vi "FPGAController_v5.1.vi"() -> ()   [LabVIEW 2015]
uses:
  Detector_Cluster.ctl
  <vilib>/Utility/miscctls.llb/LVPointTypeDef.ctl
  <vilib>/FPGAPlugInAG/PXIe-7971R/niLvFpga_Open_PXIe-7971R.vi
  <userlib>/_OpenG.lib/comparison/comparison.llb/Variant Changed__ogtk.vi
  <vilib>/Utility/error.llb/Error Cluster From Error Code.vi
  <vilib>/rvi/errors/niLvFpgaAdjustHostInterfaceError.vi
  <vilib>/FPGAPlugInAG/PXIe-7971R/niLvFpga_Close_PXIe-7971R.vi
  <vilib>/rvi/interface/nirviOpenFPGA/nirviOpenFPGA.xnode
  FPGA Bitfiles/FPGA2_FPGATarget_FPGAcode2.1_u+OfLr1fgUM.lvbitx
  <vilib>/rvi/interface/nirviReadWriteControl/nirviReadWriteControl.xnode
  Limits_In.ctl
  <vilib>/rvi/interface/nirviCloseFPGA/nirviCloseFPGA.xnode
  NiFpgaLv.dll
panel:
  in  "Trigger String 2":string="Disarm Trigger"
  in  "Trigger String 1":string="Rearm Trigger"
  in  "Tab Control":enum32{"IO/Control", "Error Management"}(tab)
  out "Trigger Armed":bool
  in  "Arm Trigger":bool
  in  "One Shot Mode":bool
  in  "Auto Threshold":bool
  in  "Sensitivity":dbl=1.2 step=0.2 format="%_3g"
  in  "Filter Thresholds":T1={"1"=887988, "2"=361992, "3"=138762, "4"=54306, "5"=41730, "6"=29358, "7"=21165}
  in  "error in (no error)":errorcluster
  out "error out":errorcluster
  out "Runtime Error":errorcluster
  out "Updating PSU":bool
  in  "stop":bool
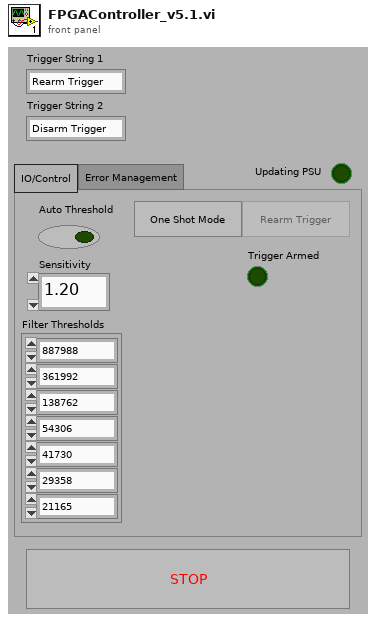
[diagram p1: front panel]
types:
  T1 = typedef "Detector_Cluster.ctl" = cluster{"1":i32, "2":i32, "3":i32, "4":i32, "5":i32, "6":i32, "7":i32}
  T2 = enum8{"Enabled", "Disabled", "Disabled and Grayed Out"}
  T3 = typedef "LVPointTypeDef.ctl" = cluster{"Horizontal":i16, "Vertical":i16}
  T4 = typedef "Limits_In.ctl" = cluster{"High Charge Limit":i16, "Low Charge Limit":i16, "High Velocity Count":i32, "Low Velocity Count":i32, "High Mass Limit":i64, "Low Mass Limit":i64}
  T5 = cluster{"1":dbl, "2":dbl, "3":dbl, "4":dbl, "5":dbl, "6":dbl, "7":dbl}
  T6 = cluster{"1":i16, "2":i16, "3":i16, "4":i16, "5":i16, "6":i16, "7":i16}
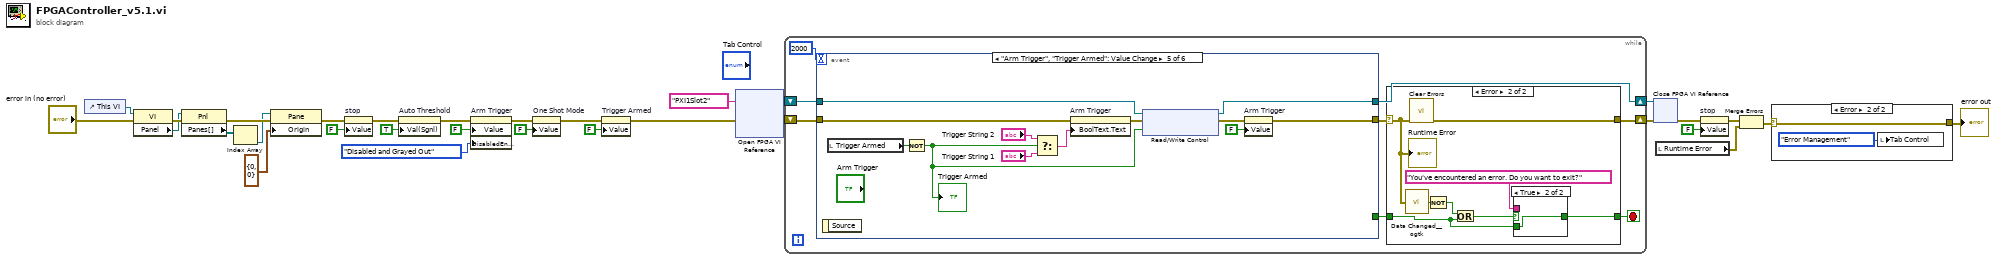
[diagram p0: block diagram]
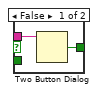
[diagram p4: hidden frame]
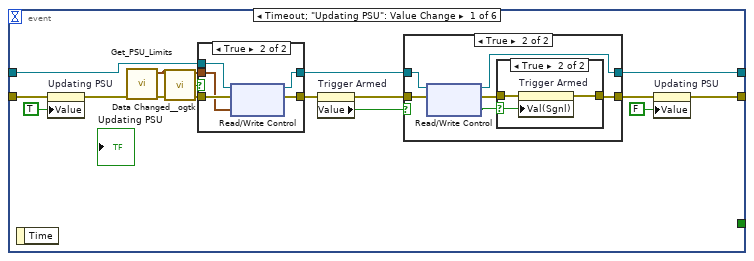
[diagram p5: hidden frame]
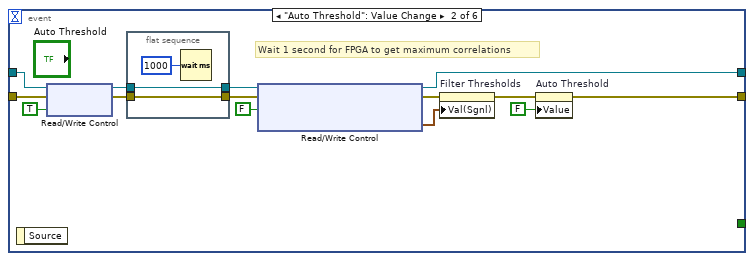
[diagram p9: hidden frame]
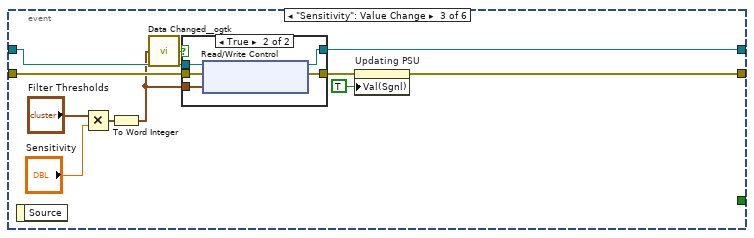
[diagram p10: hidden frame]
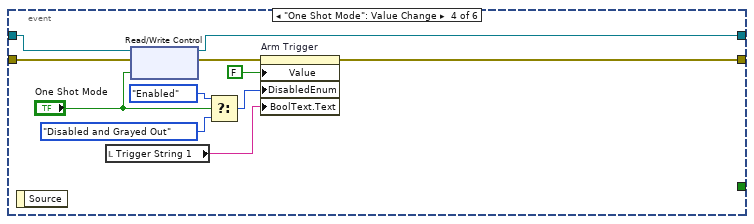
[diagram p12: hidden frame]
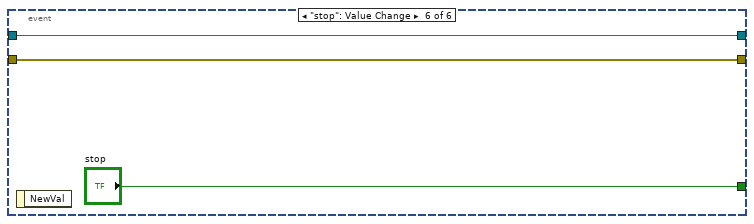
[diagram p13: hidden frame]
diagram:
  n1 = control-ref of="This VI"() -> (w31:refnum<vi>)
  n2 = property class="VI"(reference=w31, error in="error in (no error)") -> (error out=w30:errorcluster, "Panel"=w29:refnum<vi>)  [unwired: 1 out]
  n3 = property class="Pnl"(reference=w29, error in=w30) -> (error out=w28:errorcluster, "Panes[]"=w27:refnum<vi>[])  [unwired: 1 out]
  n4 = Index Array(array=w27) -> (element=w26:refnum<vi>)  [unwired: 1 in]
  n5 = property class="Pane"(reference=w26, error in=w28, "Origin"=T3 {"Horizontal"=0, "Vertical"=0}) -> (error out=w19:errorcluster)  [unwired: 1 out]
  n6 = property on="stop" class="Bool (strict)"(error in=w19, "Value"=FALSE ("stop")) -> (error out=w15:errorcluster)  [unwired: 1 in, 1 out]
  n7 = property on="Auto Threshold" class="Bool (strict)"(error in=w15, "Val(Sgnl)"=TRUE ("Value (Signaling)")) -> (error out=w7:errorcluster)  [unwired: 1 in, 1 out]
  n8 = property on="Arm Trigger" class="Bool (strict)"(error in=w7, "Value"=FALSE ("Arm Trigger"), "DisabledEnum"=T2."Disabled and Grayed Out" ("Disabled")) -> (error out=w5:errorcluster)  [unwired: 1 in, 1 out]
  n9 = property on="One Shot Mode" class="Bool (strict)"(error in=w5, "Value"=FALSE ("One Shot Mode")) -> (error out=w3:errorcluster)  [unwired: 1 in, 1 out]
  n10 = property on="Trigger Armed" class="Bool (strict)"(error in=w3, "Value"=FALSE ("Armed")) -> (error out=w1:errorcluster)  [unwired: 1 in, 1 out]
  n11 = xnode "Open FPGA VI Reference"("error in"=w1, "resource name"=tag "PXI1Slot2") -> ("FPGA VI Reference Out"=w23:refnum<k20>, "error out"=w21:errorcluster)
  n12 = while {
    shift-right: [w32] -> w20
    shift-left: w21 -> [w38]
    shift-right: [w36] -> w22
    shift-left: w23 -> [w37]
    stop <- w34 stop-if-true
    n13 = event shown="[4] \"Arm Trigger\", \"Trigger Armed\": Value Change" {
      selector: _ -> [_ _ _ _ _ _]
      dyn-events: _ -> [_ _ _ _ _ _]
      timeout: 2000 -> [_ _ _ _ _ _]
      tunnel: [_ _ _ _ _ "stop"] -> w33
      tunnel: w38 -> [w65 w98 w113 w132 w144 w146]
      tunnel: [w59 w100 w107 w124 w134 w146] -> w35
      tunnel: w37 -> [w67 w97 w114 w131 w139 w145]
      tunnel: [w54 w92 w110 w123 w138 w145] -> w36
      event Timeout; "Updating PSU": Value Change {
        n14 = event-data() -> ()  [unwired: 1 in, 1 out]
        n15 = property on="Updating PSU" class="Bool (strict)"(error in=w65, "Value"=TRUE ("Updating PSU")) -> (error out=w62:errorcluster)  [unwired: 1 in, 1 out]
        n16 = call "Get_PSU_Limits.vi"("error in (no error)"=w62) -> ("error out"=w66:errorcluster, "Limits"=w61:T4)  [unwired: 9 in]
        n17 = call-poly <userlib>:"Data Changed__ogtk.vi"("Variant"=w61) -> ("Changed"=w60:bool)
        n18 = case shown="True" w60 {
          tunnel: w67 -> [w81 w86]
          tunnel: w66 -> [w80 w85]
          tunnel: [w81 w84] -> w55
          tunnel: [w80 w83] -> w58
          tunnel: w61 -> [_ w82]
          frame False {
          }
          frame True {
            n19 = xnode "Read/Write Control"("FPGA VI Reference In"=w86, "error in"=w85, "Limits"=w82) -> ("FPGA VI Reference Out"=w84:refnum<k20>, "error out"=w83:errorcluster)
          }
        }
        n20 = property on="Trigger Armed" class="Bool (strict)"(error in=w58) -> (error out=w56:errorcluster, "Value"=w57:bool)  [unwired: 1 in, 1 out]
        n21 = case shown="True" w57 {
          tunnel: w56 -> [w68 w75]
          tunnel: w55 -> [w69 w74]
          tunnel: [w69 w73] -> w54
          tunnel: [w68 w71] -> w53
          frame False {
          }
          frame True {
            n22 = xnode "Read/Write Control"("FPGA VI Reference In"=w74, "error in"=w75) -> ("FPGA VI Reference Out"=w73:refnum<k20>, "error out"=w72:errorcluster, "Armed"=w70:bool)
            n23 = case shown="True" w70 {
              selector: w70 -> [_ w77]
              tunnel: w72 -> [w76 w79]
              tunnel: [w76 w78] -> w71
              frame False {
              }
              frame True {
                n24 = property on="Trigger Armed" class="Bool (strict)"(error in=w79, "Val(Sgnl)"=w77) -> (error out=w78:errorcluster)  [unwired: 1 in, 1 out]
              }
            }
          }
        }
        n25 = property on="Updating PSU" class="Bool (strict)"(error in=w53, "Value"=FALSE ("Updating PSU")) -> (error out=w59:errorcluster)  [unwired: 1 in, 1 out]
      }
      event "Auto Threshold": Value Change {
        # "Wait 1 second for FPGA to get maximum correlations"
        n26 = event-data() -> ()  [unwired: 1 in, 1 out]
        n27 = xnode "Read/Write Control"("FPGA VI Reference In"=w97, "error in"=w98, "Calibrate"=TRUE) -> ("FPGA VI Reference Out"=w95:refnum<k20>, "error out"=w96:errorcluster)
        n28 = flat-sequence {
          tunnel: w96 -> [w101]
          tunnel: w95 -> [w102]
          tunnel: [w102] -> w94
          tunnel: [w101] -> w93
          frame #0 {
            n29 = Wait (ms)(milliseconds to wait=u32 1000) -> ()  [unwired: 1 out]
          }
        }
        n30 = xnode "Read/Write Control"("FPGA VI Reference In"=w94, "error in"=w93, "Calibrate"=FALSE) -> ("FPGA VI Reference Out"=w92:refnum<k20>, "error out"=w88:errorcluster, "Detector 3 Max Correlations"=w89:T1)
        n31 = property on="Filter Thresholds" class="Clust (strict)"(error in=w88, "Val(Sgnl)"=w89) -> (error out=w87:errorcluster)  [unwired: 1 in, 1 out]
        n32 = property on="Auto Threshold" class="Bool (strict)"(error in=w87, "Value"=FALSE ("Auto Threshold")) -> (error out=w100:errorcluster)  [unwired: 1 in, 1 out]
      }
      event "Sensitivity": Value Change {
        n33 = event-data() -> ()  [unwired: 1 in, 1 out]
        n34 = Multiply(x="Filter Thresholds", y="Sensitivity") -> (x*y=w112:T5)
        n35 = To Word Integer(number=w112) -> (16bit integer=w104:T6)
        n36 = call-poly <userlib>:"Data Changed__ogtk.vi"("Variant"=w104) -> ("Changed"=w105:bool)
        n37 = case shown="True" w105 {
          tunnel: w114 -> [w115 w121]
          tunnel: w113 -> [w116 w120]
          tunnel: [w115 w119] -> w110
          tunnel: [w116 w118] -> w108
          tunnel: w104 -> [_ w117]
          frame False {
          }
          frame True {
            n38 = xnode "Read/Write Control"("FPGA VI Reference In"=w121, "error in"=w120, "Filter Thresholds"=w117) -> ("FPGA VI Reference Out"=w119:refnum<k20>, "error out"=w118:errorcluster)
          }
        }
        n39 = property on="Updating PSU" class="Bool (strict)"(error in=w108, "Val(Sgnl)"=TRUE ("Updating PSU")) -> (error out=w107:errorcluster)  [unwired: 1 in, 1 out]
      }
      event "One Shot Mode": Value Change {
        n40 = event-data() -> ()  [unwired: 1 in, 1 out]
        n41 = local read "Trigger String 1"() -> (w122:string)
        n42 = xnode "Read/Write Control"("FPGA VI Reference In"=w131, "error in"=w132, "One Shot"="One Shot Mode") -> ("FPGA VI Reference Out"=w123:refnum<k20>, "error out"=w129:errorcluster)
        n43 = Select(t=T2."Enabled" ("Disabled"), s="One Shot Mode", f=T2."Disabled and Grayed Out" ("Disabled")) -> (s? t:f=w127:T2)
        n44 = property on="Arm Trigger" class="Bool (strict)"(error in=w129, "Value"=FALSE ("Arm Trigger"), "DisabledEnum"=w127, "BoolText.Text"=w122) -> (error out=w124:errorcluster)  [unwired: 1 in, 1 out]
      }
      event "Arm Trigger", "Trigger Armed": Value Change {
        n45 = event-data() -> ()  [unwired: 1 in, 1 out]
        n46 = local read "Trigger Armed"() -> (w137:bool)
        n47 = Not(x=w137) -> (.not. x?=w136:bool)
        "Trigger Armed" <- w136
        n48 = Select(t="Trigger String 2", s=w136, f="Trigger String 1") -> (s? t:f=w141:string)
        n49 = property on="Arm Trigger" class="Bool (strict)"(error in=w144, "BoolText.Text"=w141) -> (error out=w140:errorcluster)  [unwired: 1 in, 1 out]
        n50 = xnode "Read/Write Control"("FPGA VI Reference In"=w139, "error in"=w140, "Reset One Shot"=w136) -> ("FPGA VI Reference Out"=w138:refnum<k20>, "error out"=w135:errorcluster)
        n51 = property on="Arm Trigger" class="Bool (strict)"(error in=w135, "Value"=FALSE ("Arm Trigger")) -> (error out=w134:errorcluster)  [unwired: 1 in, 1 out]
      }
      event "stop": Value Change {
        n52 = event-data() -> ()  [unwired: 1 in, 1 out]
      }
    }
    n53 = case shown="Error" w35 {
      selector: w35 -> [w41 w46]
      tunnel: [w41 w49] -> w32
      tunnel: [w40 w47] -> w34
      tunnel: w33 -> [w40 w42]
      frame No Error {
      }
      frame Error {
        n54 = call-poly <userlib>:"Data Changed__ogtk.vi"("Variant"=w46) -> ("Changed"=w44:bool)
        n55 = call <vilib>:"Clear Errors.vi"("error in (no error)"=w46) -> ("error out"=w49:errorcluster)  [unwired: 5 in, 1 out]
        n56 = Not(x=w44) -> (.not. x?=w43:bool)
        n57 = Or(x=w43, y=w42) -> (x .or. y?=w45:bool)
        n58 = case shown="True" w45 {
          tunnel: "You've encountered an error. Do you want to exit?" ("message") -> [w51 _]
          tunnel: [w50 w52] -> w47
          tunnel: w42 -> [_ w52]
          frame False {
            n59 = Two Button Dialog(message=w51) -> (T button?=w50:bool)  [unwired: 2 in]
          }
          frame True {
          }
        }
        "Runtime Error" <- w46
      }
    }
  }
  n60 = xnode "Close FPGA VI Reference"("FPGA VI Reference In"=w22, "error in"=w20) -> ("error out"=w16:errorcluster)
  n61 = local read "Runtime Error"() -> (w11:errorcluster)
  n62 = property on="stop" class="Bool (strict)"(error in=w16, "Value"=FALSE ("stop")) -> (error out=w12:errorcluster)  [unwired: 1 in, 1 out]
  n63 = Merge Errors(w12, w11) -> (w9:errorcluster)
  n64 = case shown="Error" w9 {
    selector: w9 -> [w148 w149]
    tunnel: [w148 w149] -> w10
    frame No Error {
    }
    frame Error {
      n65 = local write "Tab Control"(enum32{"IO/Control", "Error Management"}."Error Management" ("Tab Control")) -> ()
    }
  }
  "error out" <- w10
